vi "Dextra.vi"() -> ()   [LabVIEW 2009]
uses:
  <vilib>/Platform/TimedLoop/XDataNode/XDataNode.xnode
  <vilib>/Platform/TimedLoop/XDataNode/loadlvalarms.vi
  <vilib>/Platform/TimedLoop/XDataNode/timing_clust.ctl
  <vilib>/Platform/TimedLoop/XDataNode/nitl_modes.ctl
  <vilib>/Platform/TimedLoop/XDataNode/wakeup.ctl
  <vilib>/Platform/TimedLoop/XDataNode/XDNodeRunTimeDep.lvlib
panel:
  in  "Tab Control":enum32{"Main", "EMG", "FINGERS", "ACM", "WRIST"}(tab)
  out "Array 10":bool[](array[boolean])
  out "Array 9":bool[](array[boolean])
  out "Array 8":bool[](array[boolean])
  out "Array 7":bool[](array[boolean])
  out "Array 6":bool[](array[boolean])
  out "Array 5":bool[](array[boolean])
  out "Array 4":bool[](array[boolean])
  out "Array 3":bool[](array[boolean])
  out "Array 2":bool[](array[boolean])
  out "Rotacion":string
  out "Movement Type":string
  out "Acc Z":dbl
  out "Acc Y":dbl
  out "Acc X":dbl
  out "EMG Input":dynamicdata(graph)
  in  "Samples":i32=1000
  in  "Rate":dbl=1000.0
  in  "stop":bool
  out "Array":bool[](array[boolean])
  out "Array 1":bool[](array[boolean])
  out "EMG CH 1":dynamicdata(graph)
  out "EMG Input":dynamicdata(graph)
  in  "stop 2":bool
  in  "Rate 2":dbl=1000.0
  in  "Samples 2":i32=1000
  out "EMG CH 3":dynamicdata(graph)
  out "EMG CH 4":dynamicdata(graph)
  out "EMG CH 2":dynamicdata(graph)
  in  "stop 3":bool
  out "X0":bool
  out "X+":bool
  out "X-":bool
  out "MIN X+":dbl
  out "MAX X+":dbl
  out "MIN X-":dbl
  out "MAX X-":dbl
  in  "MIN X":dbl
  in  "MAX X":dbl
  in  "stop 4":bool
  out "ACM X":dbl
  in  "AMC RATE":dbl=1000.0
  in  "ACM SAMPLES":i32=1000
  in  "X0":dbl
  out "ACM Y":dbl
  in  "MAX Y":dbl
  in  "MIN Y":dbl
  out "MAX Y-":dbl
  out "MIN Y-":dbl
  out "MAX Y+":dbl
  out "MIN Y+":dbl
  out "Y-":bool
  out "Y+":bool
  out "Y0":bool
  in  "Y0":dbl
  out "ACM Z":dbl
  in  "MAX Z":dbl
  in  "MIN Z":dbl
  out "MAX Z-":dbl
  out "MIN Z-":dbl
  out "MAX Z+":dbl
  out "MIN Z+":dbl
  out "Z-":bool
  out "Z+":bool
  out "Z0 2":bool
  in  "Z0":dbl
  out "ACELEROMETTER INPUTS":dynamicdata(graph)
  out "ANGLE":dbl
  out "STEP":dbl
  in  "ROTATION":bool
  out "Free Run Ind":bool[](array[boolean])
  in  "STOP":bool
  in  "RUN":bool
  in  "Select Mode":u16(ring) items=["Free Run", "Manual Run"]
  in  "SPEED":dbl(knob) scale=0.0..1000.0
  # "MOVEMENT TYPE"
  # "INDICE"
  # "MEDIO"
  # "ANULAR"
  # "PULGAR"
  # "MUÑECA"
  # "HAND"
  # "ACCELEROMETTERS"
  # "FREE RUN"
  # "LEFT"
  # "RIGHT"
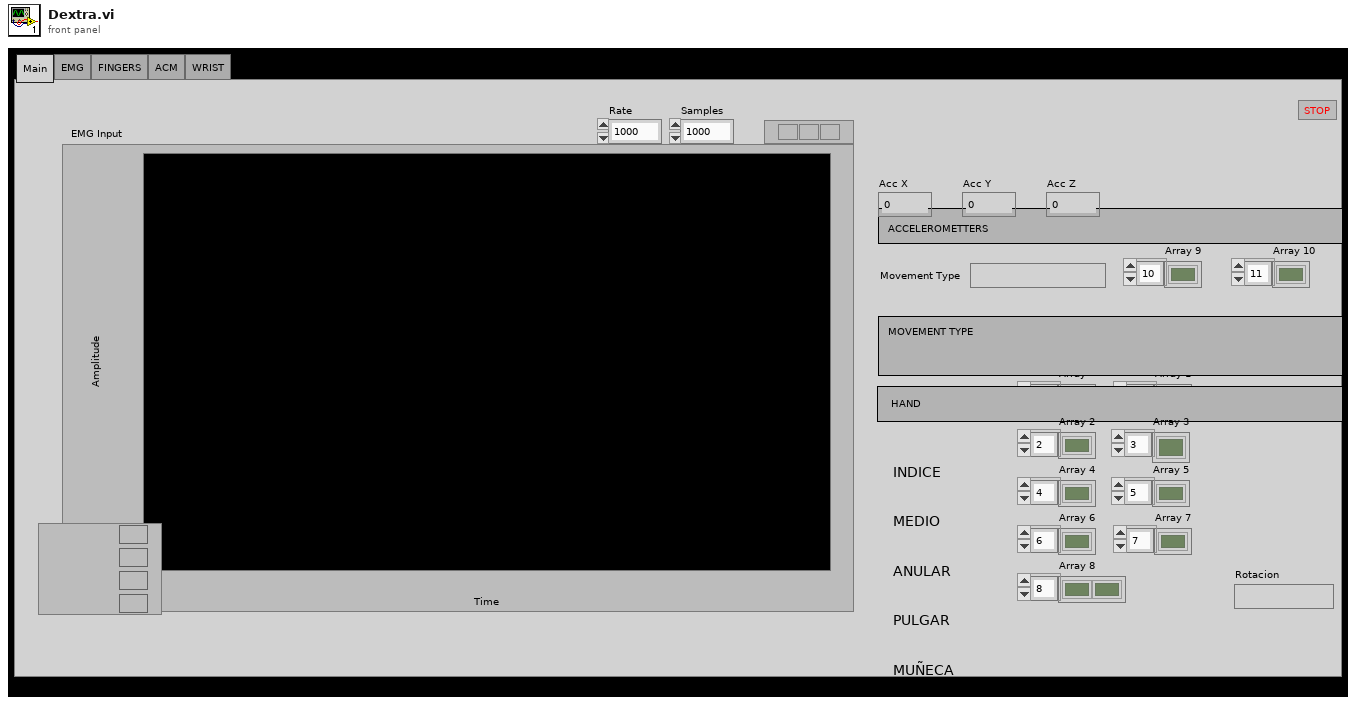
[diagram p1: front panel]
types:
  T1 = typedef "XDNodeRunTimeDep.lvlib/timing_clust.ctl" = cluster{"Expected End [f-1]":u64, "Actual End [f-1]":u64, "Finished Late? [f-1]":bool, "Expected End [i-1]":u64, "Actual End [i-1]":u64, "Finished Late? [i-1]":bool, "Expected Start [i]":u64, "Actual Start [i]":u64, "Expected Start [f]":u64, "Actual Start [f]":u64, "Source Name":string, "Structure Name":string, "Period":i64, "Deadline":i64, "Offset":i64, "Start":i64, "Priority":i32, "Timeout":i32, "Mode":T2, "Wakeup Reason":T3, "Error":errorcluster, "Source Type":string, "Secondary Source Type":string, "Global End Time":u64, "Global Start Time":u64, "Frame Duration":u64, "Iteration Duration":u64, "Assigned CPU":i32, "I/O Scan Engine Mode":u32}
  T2 = typedef "XDNodeRunTimeDep.lvlib/nitl_modes.ctl" = enum32{"No Change", "Process missed periods, maintain original phase", "Discard missed periods, maintain original phase", "Process missed periods, ignore original phase", "Discard missed periods, ignore original phase"}
  T3 = typedef "XDNodeRunTimeDep.lvlib/wakeup.ctl" = enum32{"Normal", "Aborted", "Asynchronous wakeup", "Timing source error", "Timed loop error", "Timeout"}
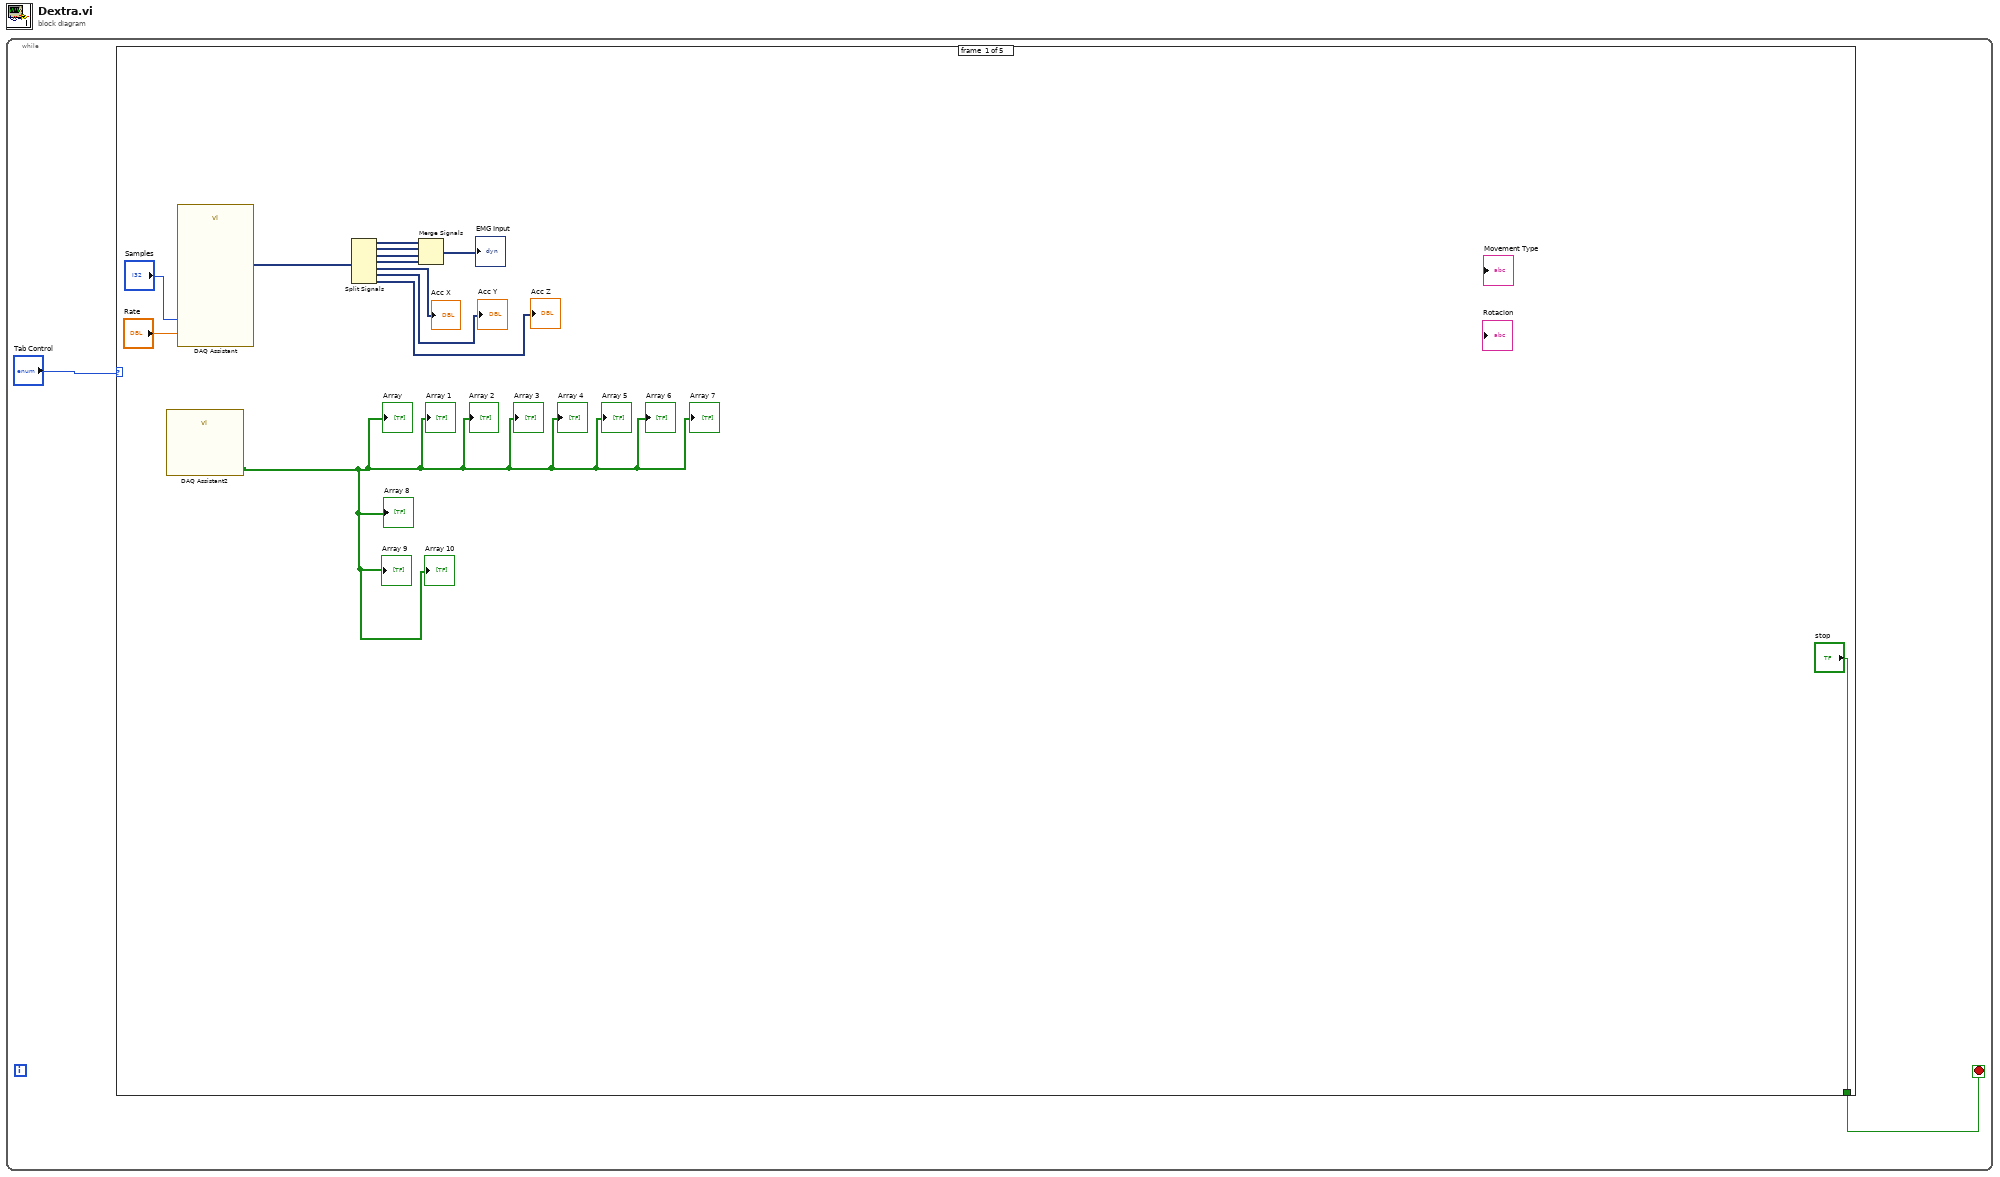
[diagram p0: block diagram]
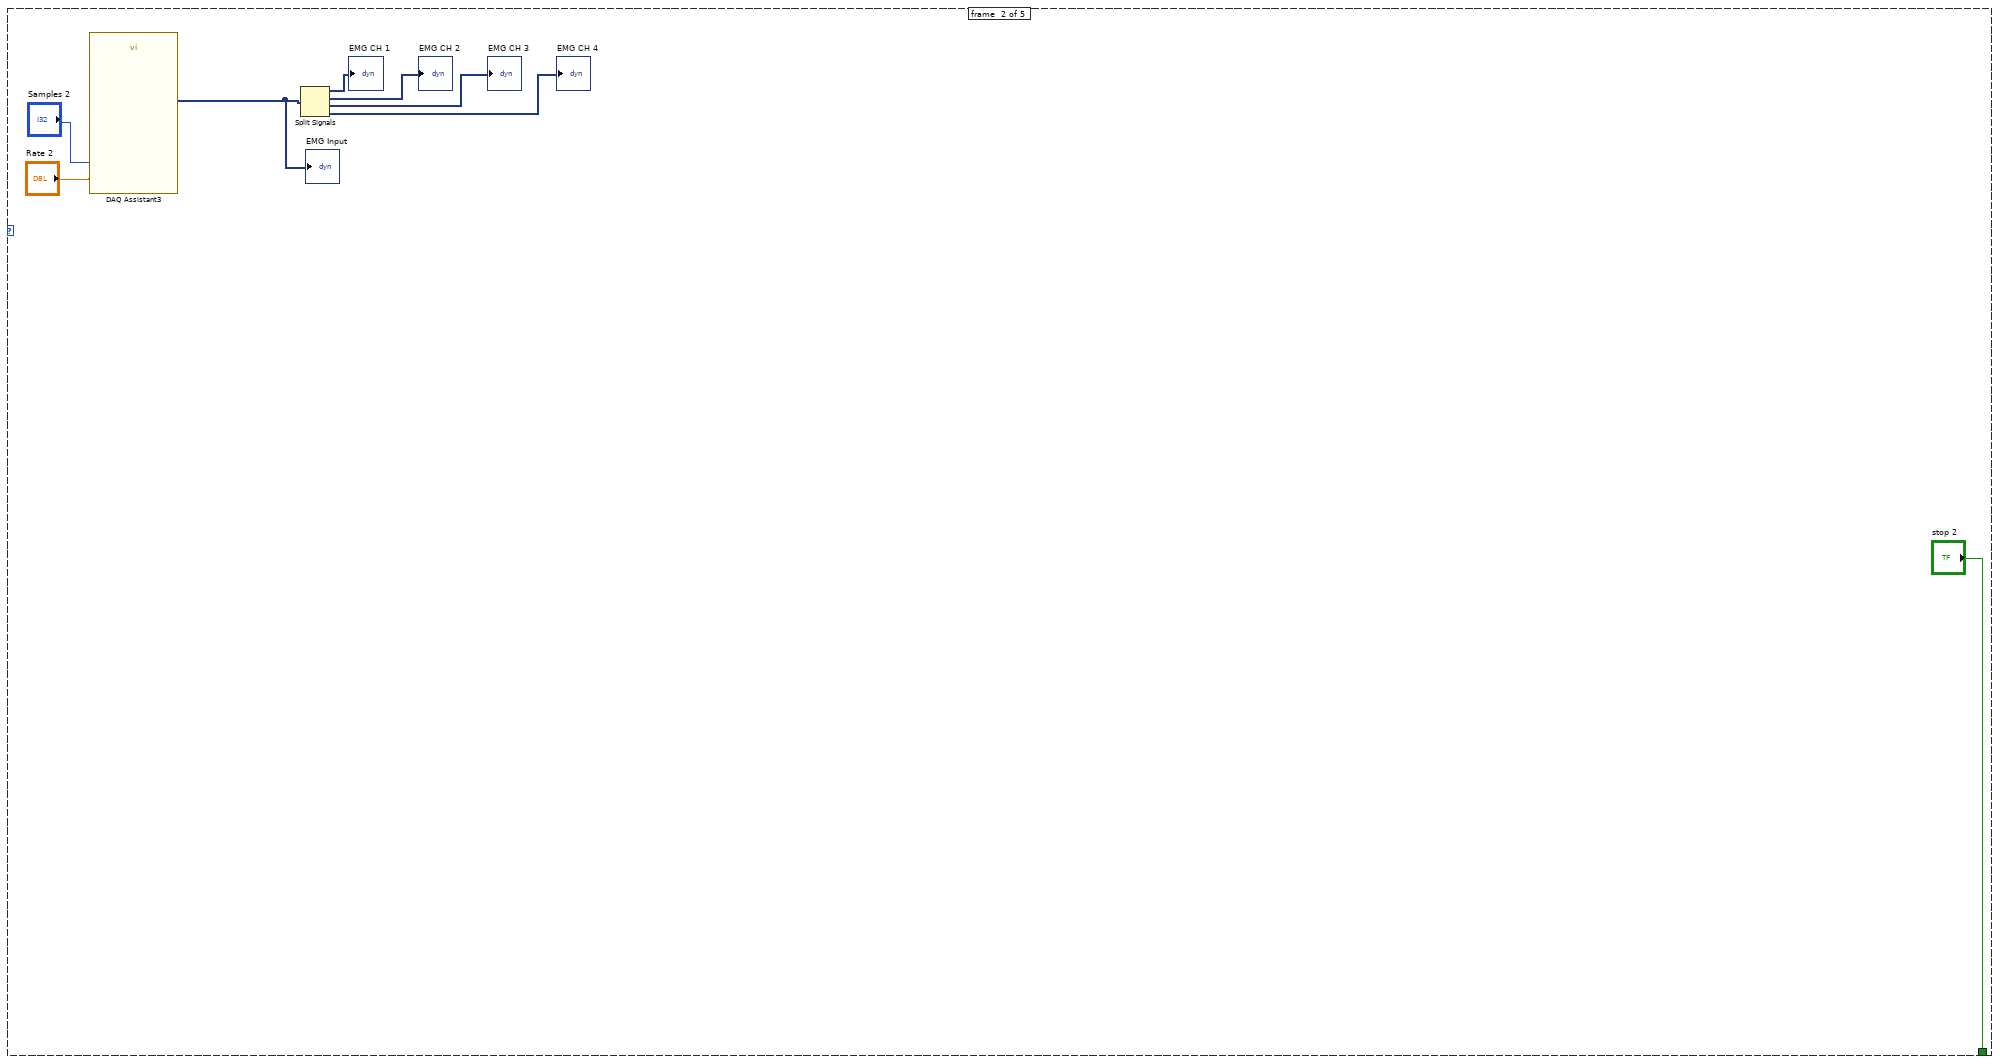
[diagram p2: hidden frame]
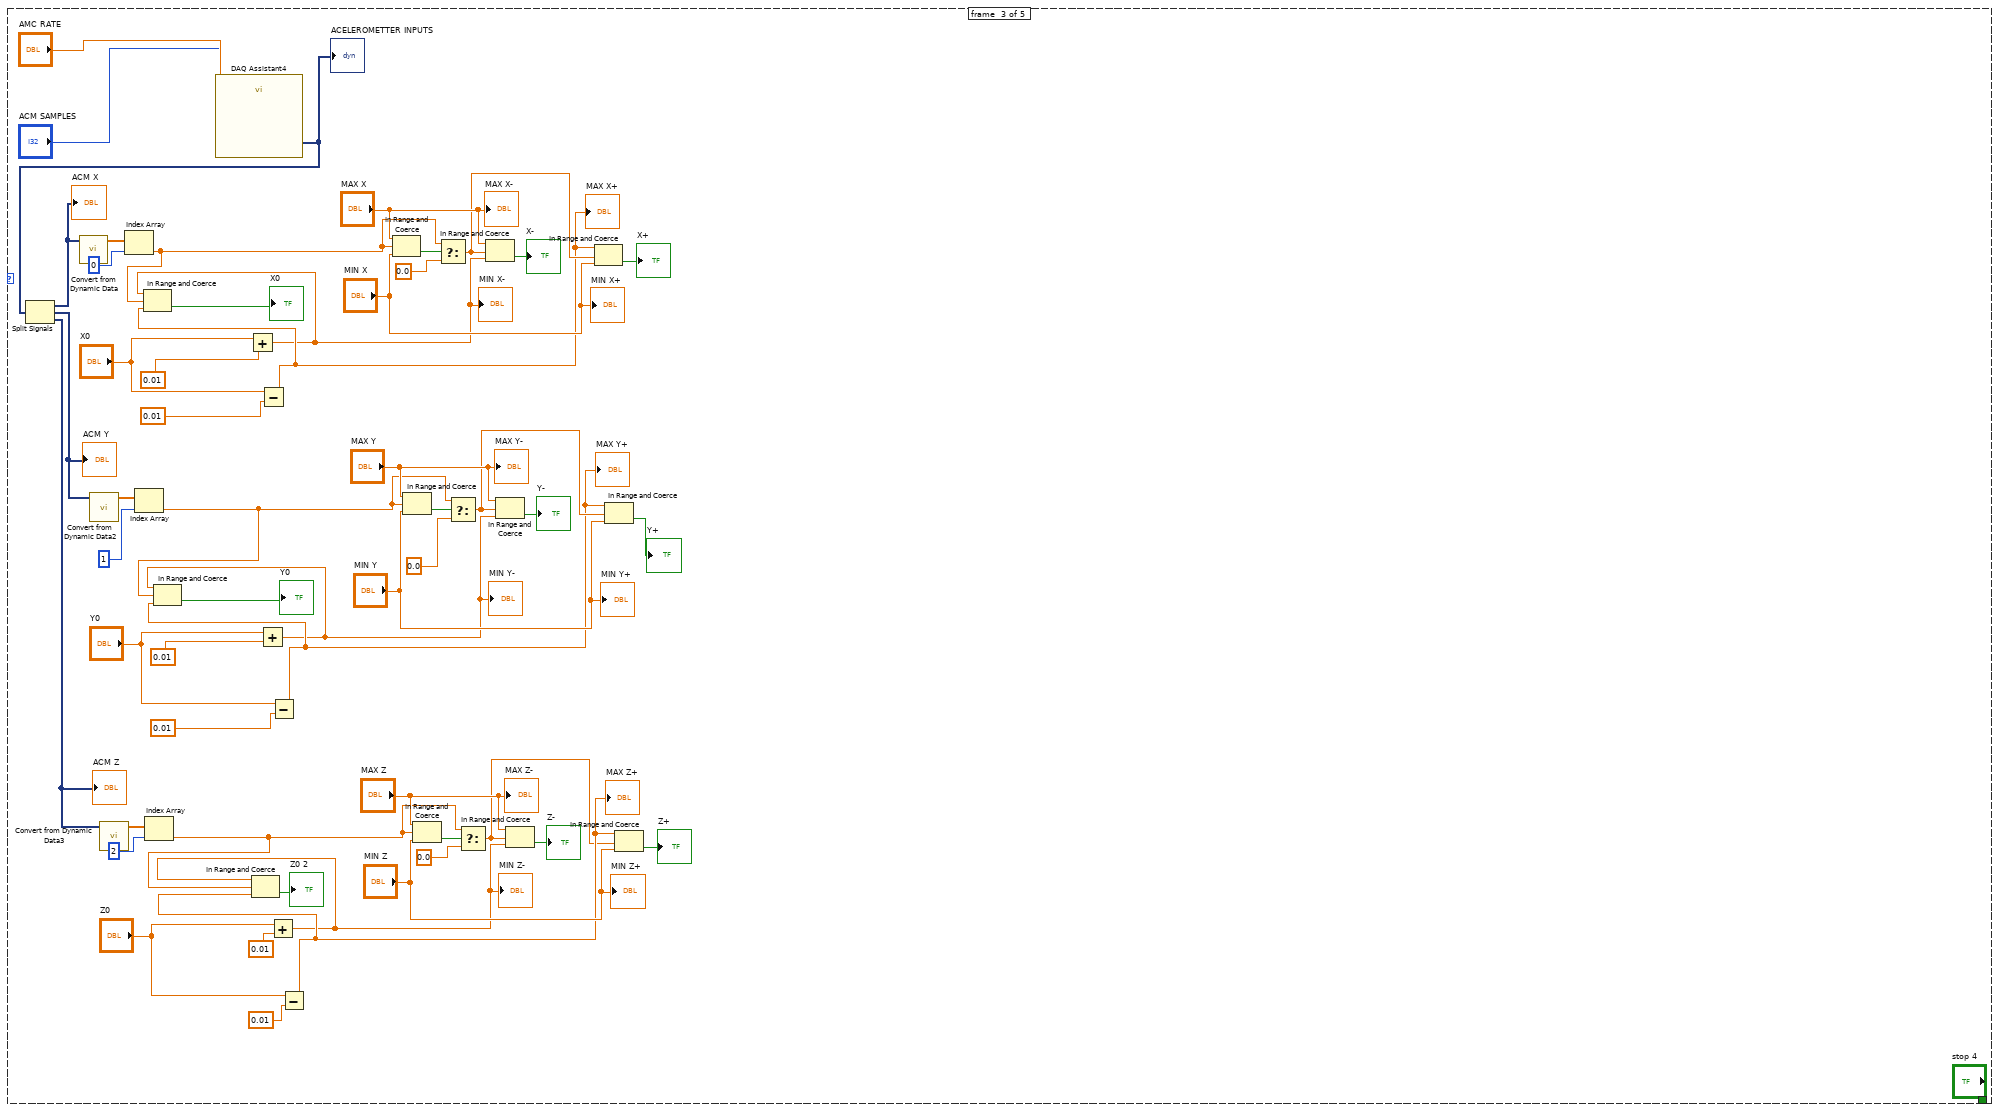
[diagram p3: hidden frame]
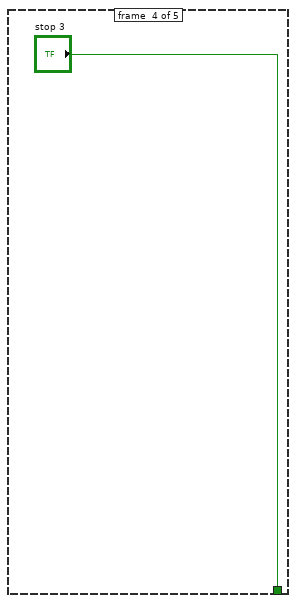
[diagram p4: hidden frame]
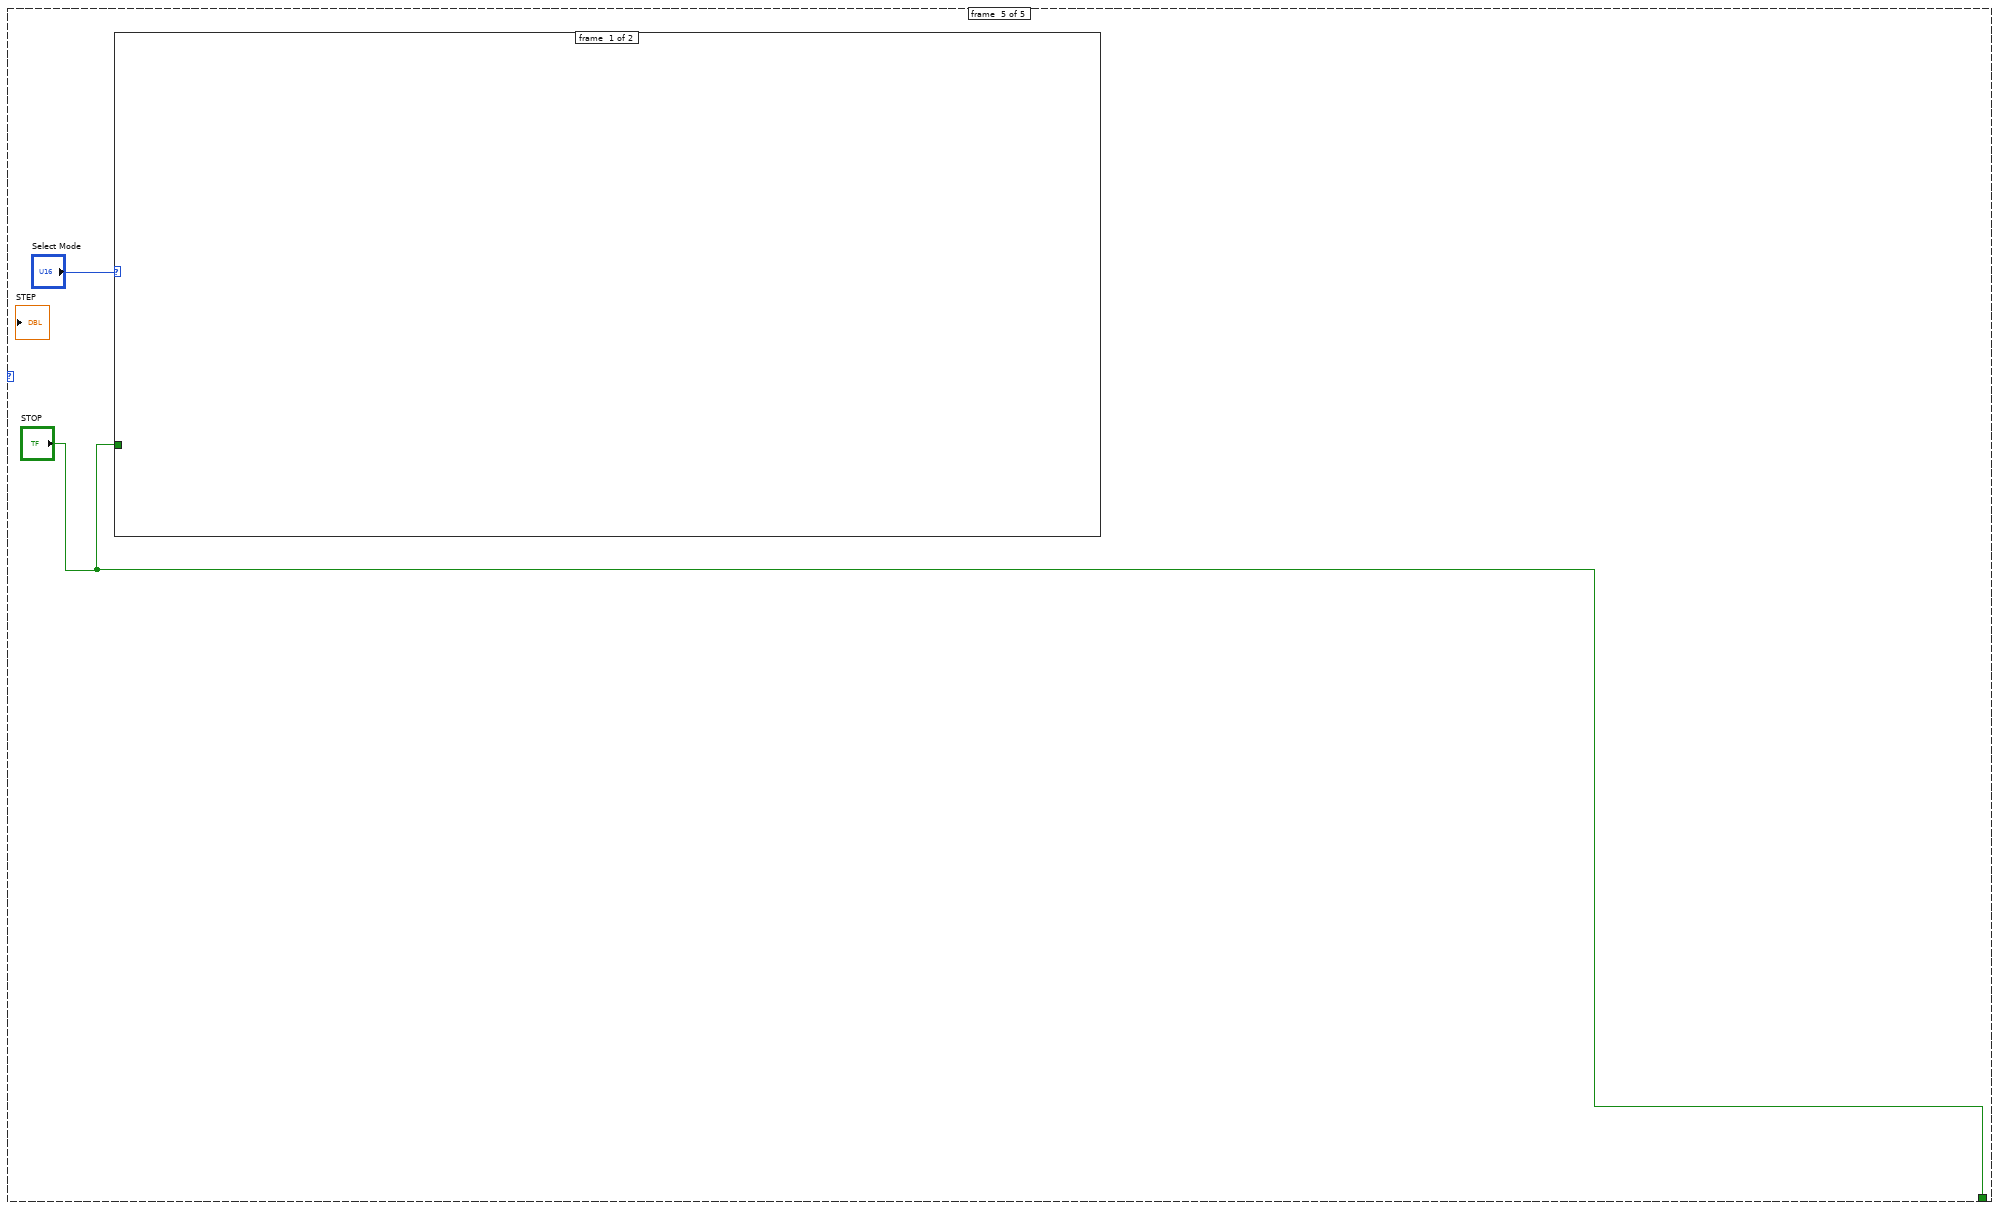
[diagram p5: hidden frame]
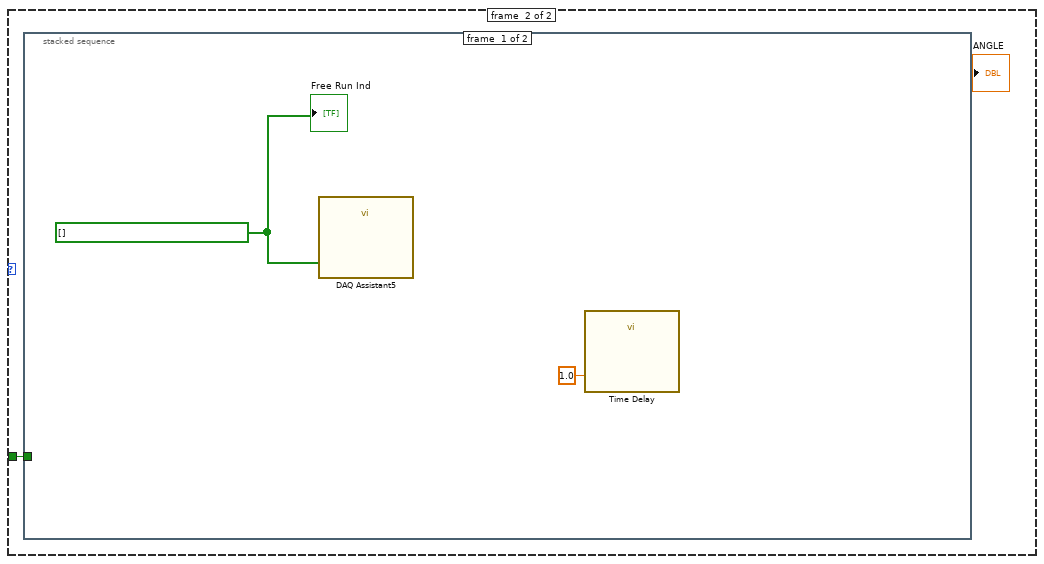
[diagram p6: hidden frame]
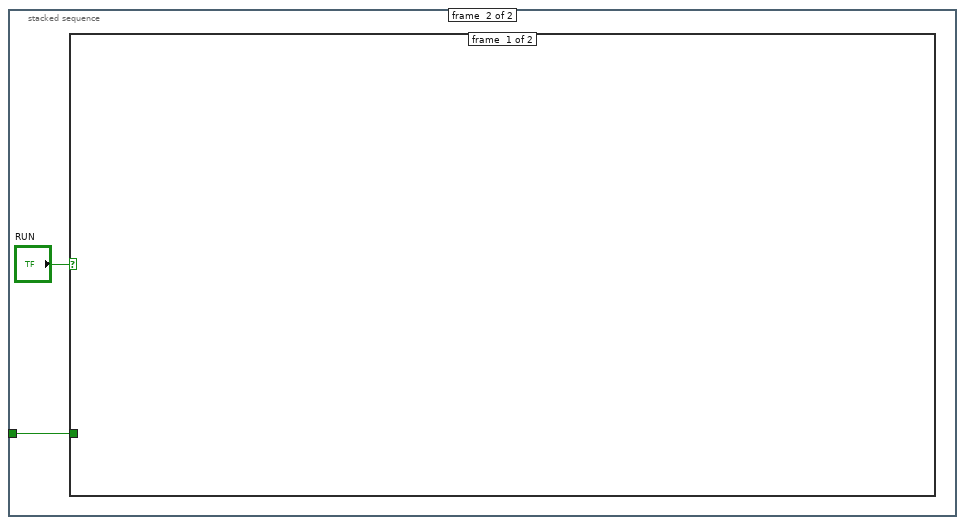
[diagram p7: hidden frame]
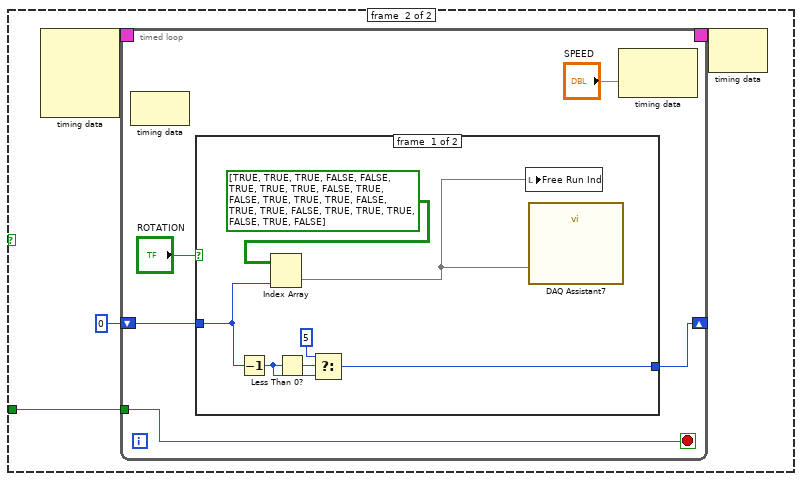
[diagram p8: hidden frame]
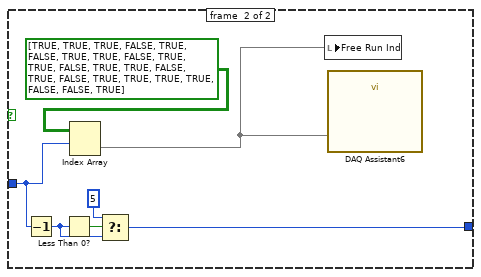
[diagram p9: hidden frame]
diagram:
  n1 = while {
    stop <- w1 stop-if-true
    n2 = case shown="\"ACM\"" "Tab Control" {
      tunnel: ["stop" "stop 2" "stop 4" "stop 3" "STOP"] -> w1
      frame #0 {
        n3 = call "DAQ Assistant2"() -> ("data"=→"Array" →"Array 1" →"Array 2" →"Array 3" →"Array 4" →"Array 5" →"Array 6" →"Array 7" →"Array 8" →"Array 9" →"Array 10":bool[])  [unwired: 17 in, 2 out]
        n4 = call "DAQ Assistant"("rate"="Rate", "number of samples"="Samples") -> ("data"=w14:dynamicdata)  [unwired: 15 in, 2 out]
        n5 = Split Signals(w14) -> (w13:dynamicdata, w11:dynamicdata, w10:dynamicdata, w9:dynamicdata, →"Acc X":dynamicdata, →"Acc Y":dynamicdata, →"Acc Z":dynamicdata)  [unwired: 7 in]
        n6 = Merge Signals(w13, w11, w10, w9) -> (→"EMG Input":dynamicdata)
      }
      frame #1 {
        n7 = call "DAQ Assistant3"("rate"="Rate 2", "number of samples"="Samples 2") -> ("data"=w16:dynamicdata)  [unwired: 15 in, 2 out]
        "EMG Input" <- w16
        n8 = Split Signals(w16) -> (→"EMG CH 1":dynamicdata, →"EMG CH 2":dynamicdata, →"EMG CH 3":dynamicdata, →"EMG CH 4":dynamicdata)  [unwired: 4 in]
      }
      frame #2 {
        n9 = call "DAQ Assistant4"("rate"="AMC RATE", "number of samples"="ACM SAMPLES") -> ("data"=w75:dynamicdata)  [unwired: 15 in, 2 out]
        "ACELEROMETTER INPUTS" <- w75
        n10 = Split Signals(w75) -> (w74:dynamicdata, w25:dynamicdata, w24:dynamicdata)  [unwired: 3 in]
        "ACM X" <- w74
        "ACM Y" <- w25
        "ACM Z" <- w24
        n11 = call "Convert from Dynamic Data"("Dynamic Data Type"=w74) -> ("Array"=w73:dbl[])  [unwired: 3 in]
        n12 = call "Convert from Dynamic Data2"("Dynamic Data Type"=w25) -> ("Array"=w57:dbl[])  [unwired: 3 in]
        n13 = call "Convert from Dynamic Data3"("Dynamic Data Type"=w24) -> ("Array"=w41:dbl[])  [unwired: 3 in]
        n14 = Index Array(array=w73, index=0) -> (element=w60:dbl)
        n15 = Index Array(array=w57, index=1) -> (element=w44:dbl)
        n16 = Index Array(array=w41, index=2) -> (element=w29:dbl)
        n17 = Add(x="X0", y=0.01) -> (x+y=w58:dbl)
        "MIN X-" <- w58
        n18 = Add(x="Y0", y=0.01) -> (x+y=w42:dbl)
        "MIN Y-" <- w42
        n19 = Subtract(x="X0", y=0.01) -> (x-y=w59:dbl)
        "MAX X+" <- w59
        n20 = In Range and Coerce(upper limit=w58, x=w60, lower limit=w59) -> (In Range?=→"X0":bool)  [unwired: 1 out]
        n21 = Add(x="Z0", y=0.01) -> (x+y=w27:dbl)
        "MIN Z-" <- w27
        n22 = Subtract(x="Y0", y=0.01) -> (x-y=w43:dbl)
        "MAX Y+" <- w43
        n23 = In Range and Coerce(upper limit=w42, x=w44, lower limit=w43) -> (In Range?=→"Y0":bool)  [unwired: 1 out]
        n24 = Subtract(x="Z0", y=0.01) -> (x-y=w28:dbl)
        "MAX Z+" <- w28
        n25 = In Range and Coerce(upper limit=w27, x=w29, lower limit=w28) -> (In Range?=→"Z0 2":bool)  [unwired: 1 out]
        n26 = In Range and Coerce(upper limit="MAX X", x=w60, lower limit="MIN X") -> (In Range?=w71:bool)  [unwired: 1 out]
        n27 = In Range and Coerce(upper limit="MAX Y", x=w44, lower limit="MIN Y") -> (In Range?=w55:bool)  [unwired: 1 out]
        n28 = In Range and Coerce(upper limit="MAX Z", x=w29, lower limit="MIN Z") -> (In Range?=w39:bool)  [unwired: 1 out]
        n29 = Select(t=w60, s=w71, f=0.0) -> (s? t:f=w67:dbl)
        n30 = Select(t=w44, s=w55, f=0.0) -> (s? t:f=w51:dbl)
        n31 = Select(t=w29, s=w39, f=0.0) -> (s? t:f=w26:dbl)
        n32 = In Range and Coerce(upper limit="MAX X", x=w67, lower limit=w58) -> (In Range?=→"X-":bool)  [unwired: 1 out]
        n33 = In Range and Coerce(upper limit="MAX Y", x=w51, lower limit=w42) -> (In Range?=→"Y-":bool)  [unwired: 1 out]
        n34 = In Range and Coerce(upper limit="MAX Z", x=w26, lower limit=w27) -> (In Range?=→"Z-":bool)  [unwired: 1 out]
        n35 = In Range and Coerce(upper limit=w59, x=w67, lower limit="MIN X") -> (In Range?=→"X+":bool)  [unwired: 1 out]
        n36 = In Range and Coerce(upper limit=w43, x=w51, lower limit="MIN Y") -> (In Range?=→"Y+":bool)  [unwired: 1 out]
        n37 = In Range and Coerce(upper limit=w28, x=w26, lower limit="MIN Z") -> (In Range?=→"Z+":bool)  [unwired: 1 out]
        "MAX X-" <- "MAX X"
        "MIN X+" <- "MIN X"
        "MAX Y-" <- "MAX Y"
        "MIN Y+" <- "MIN Y"
        "MAX Z-" <- "MAX Z"
        "MIN Z+" <- "MIN Z"
      }
      frame #3 {
      }
      frame #4 {
        n38 = case shown="1" "Select Mode" {
          tunnel: "STOP" -> [_ w82]
          frame #0 {
          }
          frame #1 {
            n39 = stacked-sequence {
              tunnel: w82 -> [_ w85]
              frame #0 {
                w83 = bool[] []
                n40 = call "DAQ Assistant5"("data"=w83) -> ()  [unwired: 17 in, 2 out]
                n41 = call "Time Delay"("Delay Time (s)"=1.0) -> ()  [unwired: 10 in, 1 out]
                "Free Run Ind" <- w83
              }
              frame #1 {
                n42 = case shown="True" "RUN" {
                  tunnel: w85 -> [_ w87]
                  frame #0 {
                  }
                  frame #1 {
                    n43 = node-c288() -> (w90:T1)  [unwired: 4 in]
                    n44 = timed-loop {
                      timing: w90 -> [_]
                      timing-out: [_] -> w89
                      shift-right: [w92] -> _
                      shift-left: 0 -> [w93]
                      tunnel: w87 -> [w91]
                      stop <- w91 stop-if-true
                      n45 = node-c288() -> ()  [unwired: 1 in, 1 out]
                      n46 = case shown="True" "ROTATION" {
                        tunnel: w93 -> [w96 w103]
                        tunnel: [w97 w104] -> w92
                        frame #0 {
                          n47 = Decrement(x=w96) -> (x-1=w98:i32)
                          n48 = Index Array(array=bool[][] [[TRUE, TRUE, TRUE, FALSE, FALSE, TRUE], [TRUE, TRUE, FALSE, TRUE, FALSE, TRUE], [TRUE, TRUE, FALSE, TRUE, TRUE, FALSE], [TRUE, TRUE, TRUE, FALSE, TRUE, FALSE]], index (col)=w96) -> (element=w101:bool[])  [unwired: 1 in]
                          n49 = Less Than 0?(x=w98) -> (x < 0?=w100:bool)
                          n50 = Select(t=5, s=w100, f=w98) -> (s? t:f=w97:i32)
                          n51 = local write "Free Run Ind"(w101) -> ()
                          n52 = call "DAQ Assistant7"("data"=w101) -> ()  [unwired: 17 in, 2 out]
                        }
                        frame #1 {
                          n53 = Decrement(x=w103) -> (x-1=w105:i32)
                          n54 = Less Than 0?(x=w105) -> (x < 0?=w107:bool)
                          n55 = Index Array(array=bool[][] [[TRUE, TRUE, TRUE, FALSE, TRUE, FALSE], [TRUE, TRUE, FALSE, TRUE, TRUE, FALSE], [TRUE, TRUE, FALSE, TRUE, FALSE, TRUE], [TRUE, TRUE, TRUE, FALSE, FALSE, TRUE]], index (row)=w103) -> (element=w108:bool[])  [unwired: 1 in]
                          n56 = Select(t=5, s=w107, f=w105) -> (s? t:f=w104:i32)
                          n57 = local write "Free Run Ind"(w108) -> ()
                          n58 = call "DAQ Assistant6"("data"=w108) -> ()  [unwired: 17 in, 2 out]
                        }
                      }
                      n59 = node-c288("SPEED") -> ()  [unwired: 1 in, 1 out]
                    }
                    n60 = node-c288(w89) -> ()  [unwired: 1 out]
                  }
                }
              }
            }
          }
        }
      }
    }
  }
